vi "Post Launch Init.vi"(8 "error in":errorcluster, 11 "Base Software in":refnum<class "Base Software.lvclass">) -> (0 "error out":errorcluster, 3 "Base Software out":refnum<class "Base Software.lvclass">, 4 "Events":T1, 6 "Self Enqueuer":refnum<class "Message Enqueuer.lvclass">)   [LabVIEW 2019, in "Base Software.lvlib" / "Main.lvlib" / "Base Software.lvclass"]
uses:
  Project/Base Software.lvclass
  C:/Users/Public/Documents/Development/builds/Engine/Engine.lvlibp/Project/Engine.lvclass
  builds/Engine/Panel.lvlibp/Panel Helper/Panel Events.ctl
  builds/Engine/Panel.lvlibp/Panel Helper/Events.ctl
  builds/Engine/Engine.lvlibp/Custom Controls/Engine Events.ctl
  builds/Engine/Engine.lvlibp/Custom Controls/System Events.ctl
  builds/Engine/Engine.lvlibp/Custom Controls/System Status.ctl
  builds/Engine/Engine.lvlibp/Custom Controls/Manual Events.ctl
  builds/Engine/Engine.lvlibp/Custom Controls/UUT_Events.ctl
  builds/Engine/Engine.lvlibp/Custom Controls/Interface Events.ctl
  builds/Engine/Actor Framework.lvlibp/1abvi3w/vi.lib/ActorFramework/Message Enqueuer/Message Enqueuer.lvclass
  Project/Base Software.lvclass/Base Software.ctl
  Accessors/StateMachine/Write State.vi
  GUI Support/State Machine Logic/Refresh State.vi
  builds/Engine/Engine.lvlibp/Accessors/Read Events.vi
  builds/Engine/Panel Manager.lvlibp/Panel Actor/Panel Actor.lvclass
  builds/Engine/Engine.lvlibp/Project/Engine.lvclass
  C:/Users/Public/Documents/Development/builds/Engine/Panel Manager.lvlibp/Panel Actor/Panel Actor.lvclass
  builds/Engine/Panel.lvlibp/Panel Helper/Panel Helper.lvclass
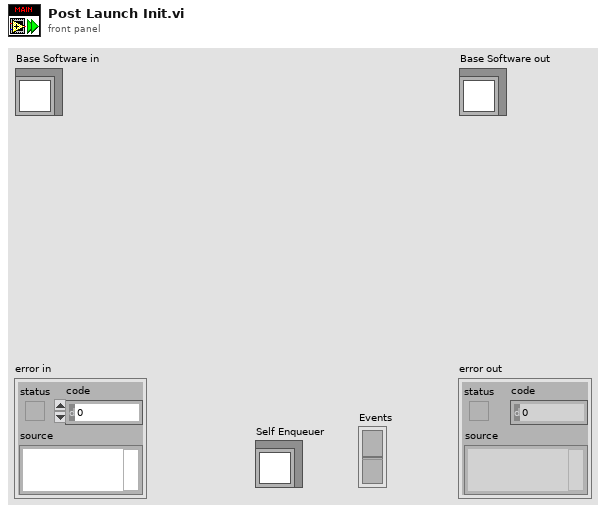
[diagram p1: front panel]
types:
  T1 = cluster{"Pnl Actor":refnum<event-registration>, "Event Registration Refnum":refnum<event-registration>}
  T2 = typedef "Engine.lvlibp/Engine.lvclass/System Status.ctl" = enum16{"Logged Off", "UUT_Info_Missing", "Idle", "Error", "Warning", "Loading", "Config", "Manual", "Automation", "Report_View", "Previous"}
  T3 = typedef "Engine.lvlibp/Engine.lvclass/Engine Events.ctl" = cluster{"System Event":T4, "Manual":T5, "UUT":T6, "Interface Events":T7}
  T4 = typedef "Engine.lvlibp/Engine.lvclass/System Events.ctl" = cluster{"Fault Event":refnum<user-event>, "SystemStatus Event":refnum<user-event>, "Automation":refnum<user-event>}
  T5 = typedef "Engine.lvlibp/Engine.lvclass/Manual Events.ctl" = cluster{"QuickStart Event":refnum<user-event>, "SafeBTE Event":refnum<user-event>, "TogglePower Event":refnum<user-event>, "Change Instrument Event":refnum<user-event>, "Toggle Launch Event":refnum<user-event>, "UUTSupply":refnum<user-event>}
  T6 = typedef "Engine.lvlibp/Engine.lvclass/UUT_Events.ctl" = cluster{"UUT_Name":refnum<user-event>, "Test_Name":refnum<user-event>, "Test_Operator":refnum<user-event>, "Test_Witness":refnum<user-event>, "Pedigree_Event":refnum<user-event>}
  T7 = typedef "Engine.lvlibp/Engine.lvclass/Interface Events.ctl" = cluster{"Interface_Command":refnum<user-event>, "Telemetry_Descriptor":refnum<user-event>, "AsynchTLM_Descriptor":refnum<user-event>}
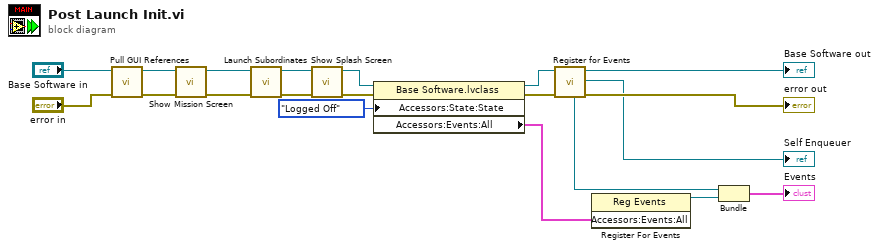
[diagram p0: block diagram]
diagram:
  n1 = call "Pull GUI References.vi"("error in"="error in", "Base Software in"="Base Software in") -> ("error out"=w3:errorcluster, "Base Software out"=w4:refnum<class "Base Software.lvclass">)  [unwired: 8 in]
  n2 = call "Show Mission Screen.vi"("error in"=w3, "Base Software in"=w4) -> ("error out"=w2:errorcluster, "Base Software out"=w1:refnum<class "Base Software.lvclass">)  [unwired: 8 in]
  n3 = call "Launch Subordinates.vi"("error in"=w2, "Base Software in"=w1) -> ("error out"=w17:errorcluster, "Base Software out"=w18:refnum<class "Base Software.lvclass">)  [unwired: 8 in]
  n4 = call "Show Splash Screen.vi"("error in"=w17, "Base Software in"=w18) -> ("error out"=w14:errorcluster, "Base Software out"=w16:refnum<class "Base Software.lvclass">)  [unwired: 8 in]
  n5 = property class="Base Software.lvclass"(reference=w16, error in=w14, "Accessors:State:State"=System_Status."Logged Off" ("Base:StateMachine:State")) -> (reference out=w15:refnum<class "Base Software.lvclass">, error out=w13:errorcluster, "Accessors:Events:All"=w12:T3)
  n6 = call "Register for Events.vi"("Error In"=w13, "Panel Actor in"=w15) -> ("Error Out"=→"error out":errorcluster, "Panel Actor out"=→"Base Software out":refnum<class "Base Software.lvclass">, "Pnl Actor"=w10:refnum<event-registration>, "Self Enqueuer"=→"Self Enqueuer":refnum<class "Message Enqueuer.lvclass">)  [unwired: 6 in]
  n7 = register-events(w12) -> (reference out=w11:refnum<event-registration>)  [unwired: 2 in, 1 out]
  n8 = Bundle("Pnl Actor"=w10, "Event Registration Refnum"=w11) -> (→"Events":T1)  [unwired: 1 in]
